vi "_File Server Simulation.vi"(2 "ErrorIn":errorcluster, 3 "FileCommand":T1) -> (0 "ErrorOut":errorcluster, 1 "DataArray":i32[](array[numeric]))   [LabVIEW 2015]
doc: "This vi maintains a datalog file for plate positions in motor steps.\nEach datalog record consists of the following data members:\nData/time in secs from 12am 1/1/1904.\nHorizontal motor steps\nVertical motor steps\nAll numbers are stored as 8-byte doubles."
uses:
  Type/_File Command.ctl
  Type/_Log Command.ctl
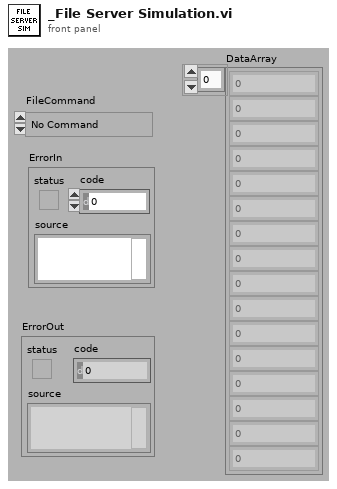
[diagram p1: front panel]
types:
  T1 = typedef "_File Command.ctl" = enum16{"No Command", "Open", "Open Read", "Write", "Get Spectrum", "Close"}
  T2 = typedef "_Log Command.ctl" = enum16{"No Command", "Open", "Read", "Write", "Close", "Check Size"}
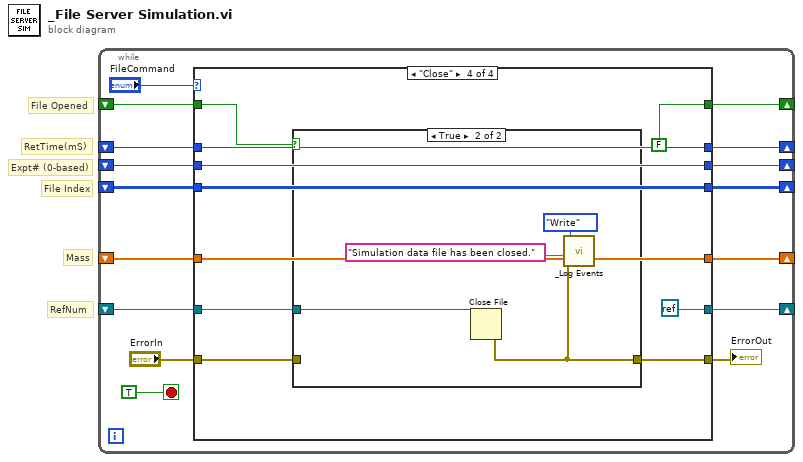
[diagram p0: block diagram]
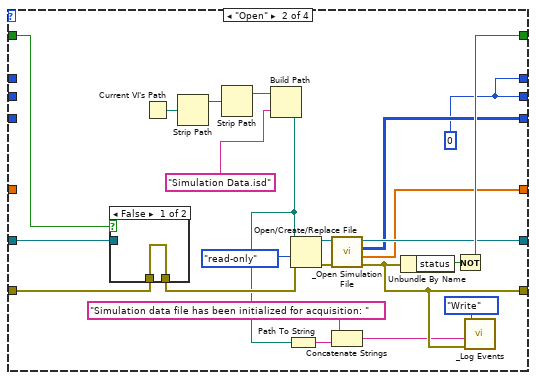
[diagram p3: hidden frame]
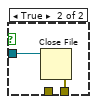
[diagram p4: hidden frame]
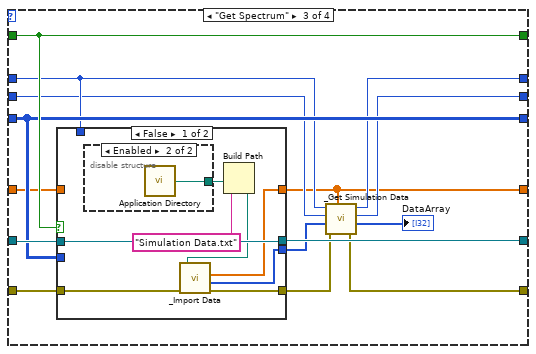
[diagram p5: hidden frame]
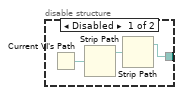
[diagram p6: hidden frame]
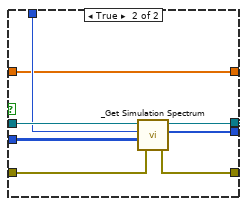
[diagram p7: hidden frame]
diagram:
  # "Expt# (0-based)"
  # "RetTime(mS)"
  # "Mass"
  # "File Index"
  # "File Opened"
  # "RefNum"
  n1 = while {
    shift-left: _ -> [w6]
    shift-right: [w12] -> _
    shift-left: _ -> [w13]
    shift-right: [w14] -> _
    shift-right: [w10] -> _
    shift-left: _ -> [w9]
    shift-right: [w8] -> _
    shift-left: _ -> [w7]
    shift-right: [w5] -> _
    shift-left: _ -> [w3]
    shift-right: [w4] -> _
    shift-left: _ -> [w2]
    stop <- TRUE stop-if-true
    n2 = case shown="\"Close\"" "FileCommand" {
      tunnel: [w23 w37 w63 refnum<k0> refnum] -> w14
      tunnel: w13 -> [w23 w43 w64 w92]
      tunnel: [w22 w45 w62 FALSE ("Record")] -> w12
      tunnel: w6 -> [w22 w44 w62 w93]
      tunnel: "ErrorIn" -> [w21 w42 w61 w91]
      tunnel: [w21 w28 w53 w90] -> w1
      tunnel: [w20 w36 w60 w88] -> w10
      tunnel: w9 -> [w20 _ w60 w88]
      tunnel: [w19 w32 w50 w87] -> w8
      tunnel: w7 -> [w19 _ w51 w87]
      tunnel: [w18 w31 w56 w86] -> w5
      tunnel: [w17 w31 w54 w85] -> w4
      tunnel: w3 -> [w18 _ w57 w86]
      tunnel: w2 -> [w17 _ w55 w85]
      frame "No Command", Default {
      }
      frame "Open" {
        w31 = 0
        n3 = case shown="False" w44 {
          tunnel: w43 -> [_ w49]
          tunnel: [w47 w48] -> w41
          tunnel: w42 -> [w47 _]
          frame False {
          }
          frame True {
            n4 = Close File(refnum=w49) -> (error out=w48:errorcluster)  [unwired: 1 in, 1 out]
          }
        }
        n5 = Current VI's Path() -> (path=w35:path)
        n6 = Strip Path(path=w35) -> (stripped path=w34:path)  [unwired: 1 out]
        n7 = Strip Path(path=w34) -> (stripped path=w33:path)  [unwired: 1 out]
        n8 = Build Path(base path=w33, name or relative path="Simulation Data.isd") -> (appended path=w27:path)
        n9 = Path To String(path=w27) -> (string=w26:string)
        n10 = Open/Create/Replace File(file path (use dialog)=w27, error in=w41, access (0:read/write)=enum16{"read/write", "read-only", "write-only"}."read-only") -> (refnum out=w39:refnum<file>, error out=w38:errorcluster)  [unwired: 1 in, 3 out]
        n11 = call "_Open Simulation File.vi"("ErrorIn"=w38, "FileRefIn"=w39) -> ("ErrorOut"=w28:errorcluster, "Mass"=w32:dbl[], "Index Array"=w36:i64[][], "FileRefOut"=w37:refnum<file>)  [unwired: 3 in, 3 out]
        n12 = Concatenate Strings("Simulation data file has been initialized for acquisition: ", w26) -> (w24:string)
        n13 = Unbundle By Name(w28) -> ("status"=w46:bool)
        n14 = Not(x=w46) -> (.not. x?=w45:bool)
        n15 = call "_Log Events.vi"("error in (no error)"=w28, "Event"=w24, "Log Command"=_Log_Command."Write" ("File Command")) -> ()  [unwired: 5 in, 2 out]
      }
      frame "Get Spectrum" {
        n16 = case shown="False" w62 {
          tunnel: w64 -> [w72 w84]
          tunnel: [w72 w83] -> w63
          tunnel: w61 -> [w69 w82]
          tunnel: [w68 w81] -> w59
          tunnel: w60 -> [_ w80]
          tunnel: [w65 w79] -> w58
          tunnel: w57 -> [_ w78]
          tunnel: [w66 w77] -> w50
          tunnel: w51 -> [_ w77]
          frame False {
            n17 = disable-structure shown="Enabled" {
              disable-tunnel: [w73 w76] -> w71
              frame Disabled {
                n18 = Current VI's Path() -> (path=w75:path)
                n19 = Strip Path(path=w75) -> (stripped path=w74:path)  [unwired: 1 out]
                n20 = Strip Path(path=w74) -> (stripped path=w73:path)  [unwired: 1 out]
              }
              frame Enabled {
                n21 = call <vilib>:"Application Directory.vi"() -> ("Application Directory"=w76:path)
              }
            }
            n22 = Build Path(base path=w71, name or relative path="Simulation Data.txt") -> (appended path=w67:path)
            n23 = call "_Import Data.vi"("error in (no error)"=w69, "file path (dialog if empty)"=w67) -> ("error out"=w68:errorcluster, "Spectrum"=w65:i32[], "Masses"=w66:dbl[])  [unwired: 2 in, 1 out]
          }
          frame True {
            n24 = call "_Get Simulation Spectrum.vi"("ErrorIn"=w82, "Index Array"=w80, "RetTime(mS)"=w78, "FileRefIn"=w84) -> ("ErrorOut"=w81:errorcluster, "Spectrum"=w79:i32[], "FileRefOut"=w83:refnum<file>)  [unwired: 1 out]
          }
        }
        n25 = call "_Get Simulation Data.vi"("SimulationMass"=w50, "ErrorIn"=w59, "SimulationSpectrum"=w58, "CurrentExpt#"=w55, "CurrentRetTime"=w57) -> ("ErrorOut"=w53:errorcluster, "DataArray"=→"DataArray":i32[], "NextExpt#"=w54:i32, "NextRetTime"=w56:i32)
      }
      frame "Close" {
        n26 = case shown="True" w93 {
          tunnel: w92 -> [_ w99]
          tunnel: w91 -> [w95 _]
          tunnel: [w95 w96] -> w90
          frame False {
          }
          frame True {
            n27 = Close File(refnum=w99) -> (error out=w96:errorcluster)  [unwired: 1 in, 1 out]
            n28 = call "_Log Events.vi"("error in (no error)"=w96, "Event"="Simulation data file has been closed.", "Log Command"=_Log_Command."Write" ("File Command")) -> ()  [unwired: 5 in, 2 out]
          }
        }
      }
    }
    "ErrorOut" <- w1
  }
